vi "Write CSV File.vi"(8 "error in":errorcluster, 10 "Data":dbl[][](array[numeric]) format="%0.2f", 11 "File Path":path) -> (0 "error out":errorcluster)   [LabVIEW 2021]
uses:
  <vilib>/Utility/file.llb/Write Delimited Spreadsheet (DBL).vi
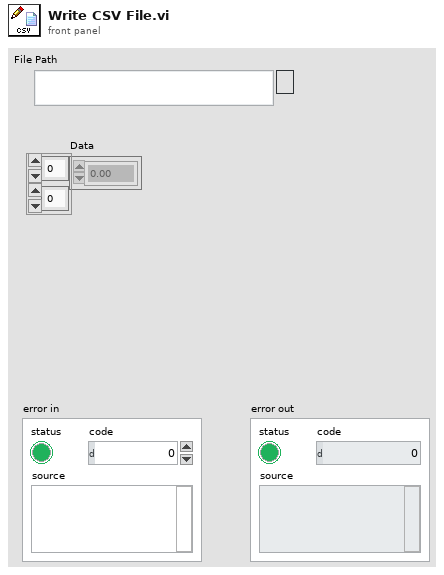
[diagram p1: front panel]
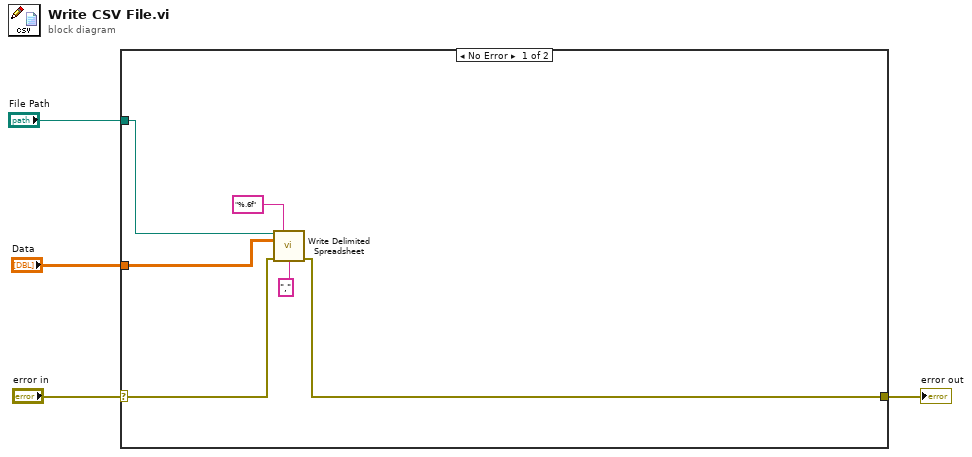
[diagram p0: block diagram]
diagram:
  n1 = case shown="No Error" "error in" {
    selector: "error in" -> [w8 w11]
    tunnel: [w7 w11] -> w3
    tunnel: "File Path" -> [w10 _]
    tunnel: "Data" -> [w9 _]
    frame No Error {
      n2 = call-poly <vilib>:"Write Delimited Spreadsheet.vi"("file path (dialog if empty)"=w10, "format (%.3f)"="%.6f", "2D data"=w9, "error in (no error)"=w8, "delimiter (\\t)"="," ("delimiter (\\t)")) -> ("error out"=w7:errorcluster)  [unwired: 9 in, 1 out]
    }
    frame Error {
    }
  }
  "error out" <- w3
